vi "thcd_400_control_1.vi"() -> ()   [LabVIEW 2019]
uses:
  thcd_controls/ctrl_chn_thcd.ctl
  thcd_controls/ctrl_sms_thcd.ctl
  <vilib>/Utility/file.llb/Write Delimited Spreadsheet (DBL).vi
  thcd_commands/thcd_set_samp.vi
panel:
  out "Sensor data":cluster{cluster{"X":dbl, "Y":dbl}[]}[](graph)
  out "thcd_st":bool
  out "thcd_res_msg":string
  in  "thcd_val":dbl min=0.0 max=100.0 step=1.0 format="%#.6g"
  in  "milliseconds to wait":u32
  out "thcd_res_4":T2
  out "thcd_res_3":T2
  out "thcd_res_2":T2
  out "thcd_res_1":T2
  in  "getstat":bool
  in  "set":bool
  in  "read":bool
  out "res_val 3":dbl
  out "res_val 2":dbl
  out "res_val":dbl
  in  "Baud_rate":u32(ring)=19200 items=["9.6KHz"=9600, "19.2KHz"=19200]
  in  "thcd_visa":refnum<visa-resource-name>
  in  "Init Devices":bool
  in  "Exit":bool
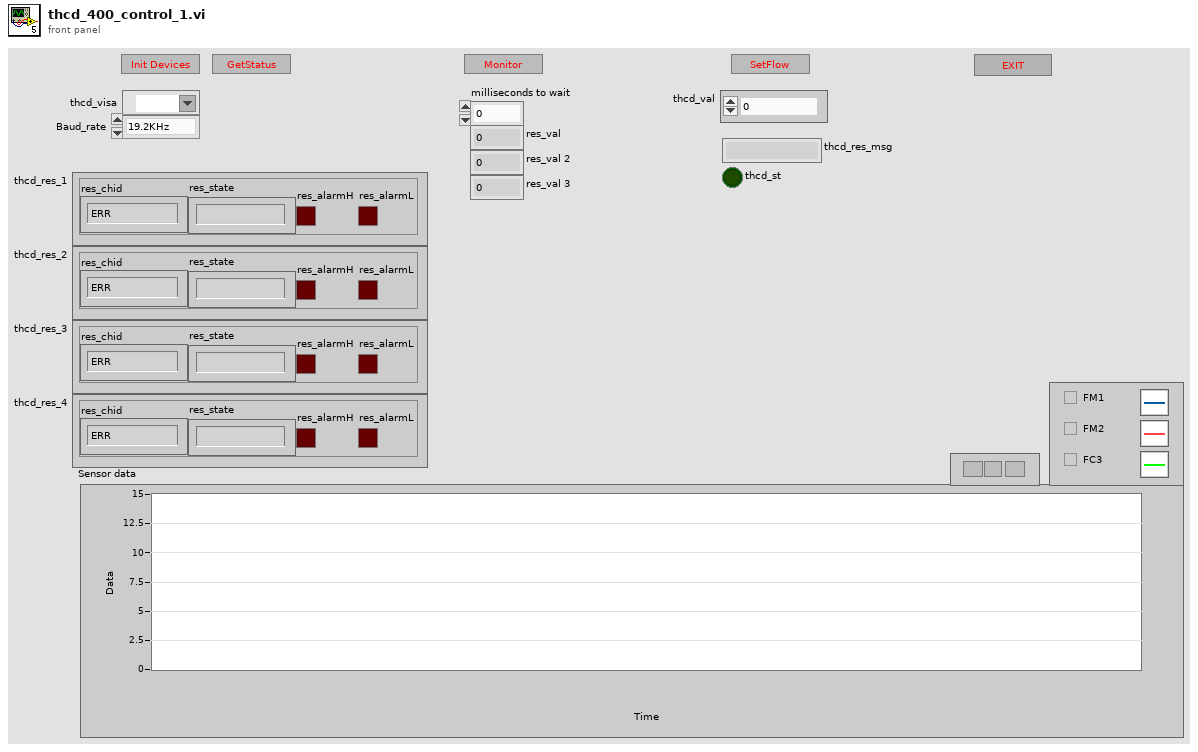
[diagram p1: front panel]
types:
  T1 = typedef "ctrl_chn_thcd.ctl" = enum8{"ERR", "1", "2", "3", "4"}
  T2 = cluster{"res_chid":T1, "res_state":string, "res_alarmH":bool, "res_alarmL":bool}
  T3 = typedef "ctrl_sms_thcd.ctl" = enum16{"idle", "init", "exit", "read", "set", "getstat"}
  T4 = enum16{"SetPoint", "AlarmH", "AlarmL", "Multiplier", "CalibValue"}
  T5 = cluster{"res_chid":T1, "res_val":dbl, "res_uom":string, "res_gid":string}[]
  T6 = cluster{"res_chid":T1, "res_val":dbl, "res_uom":string, "res_gid":string}
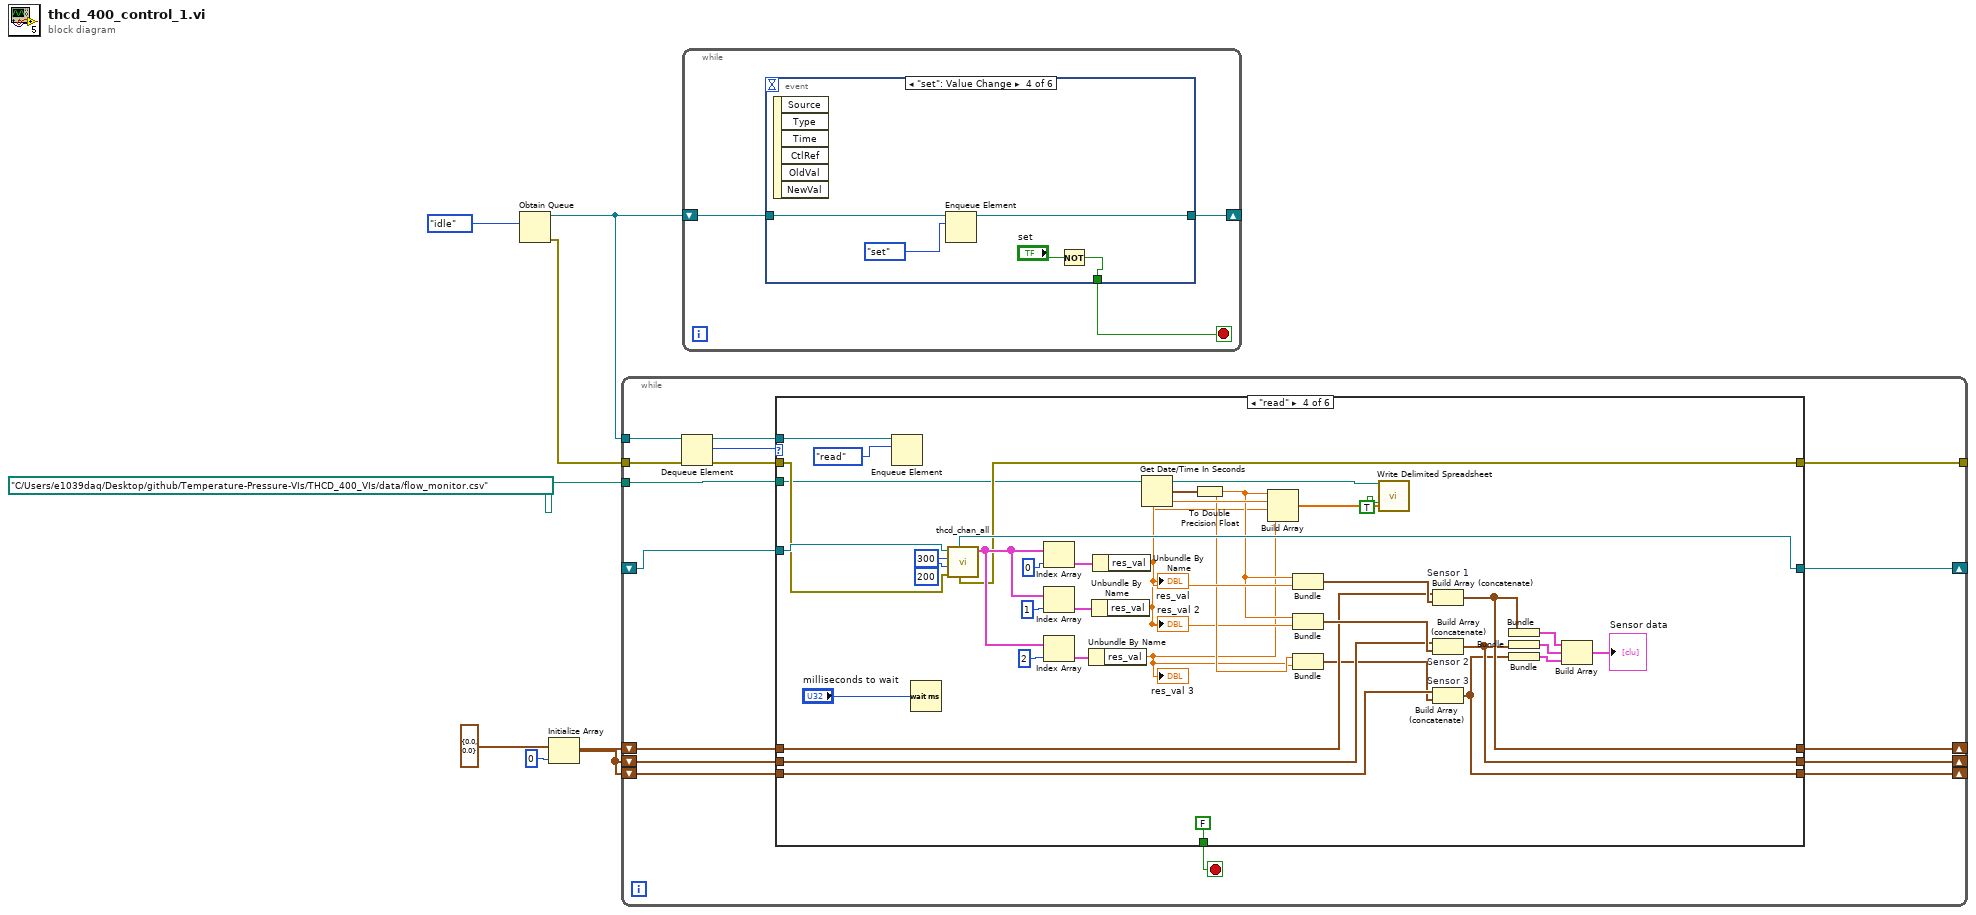
[diagram p0: block diagram]
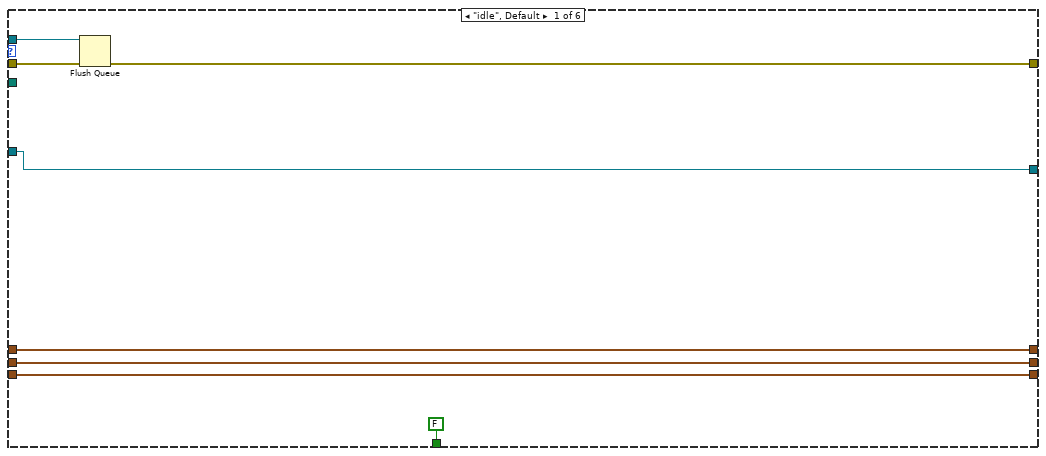
[diagram p2: hidden frame]
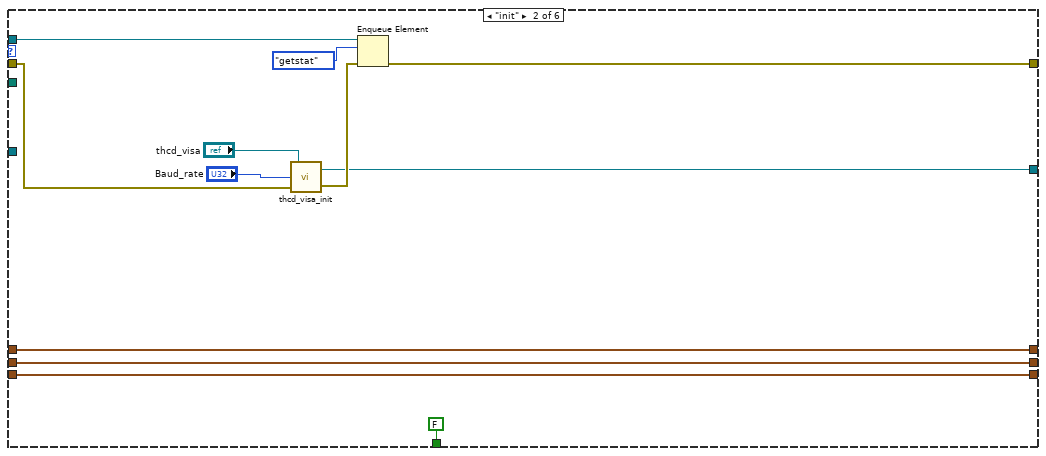
[diagram p3: hidden frame]
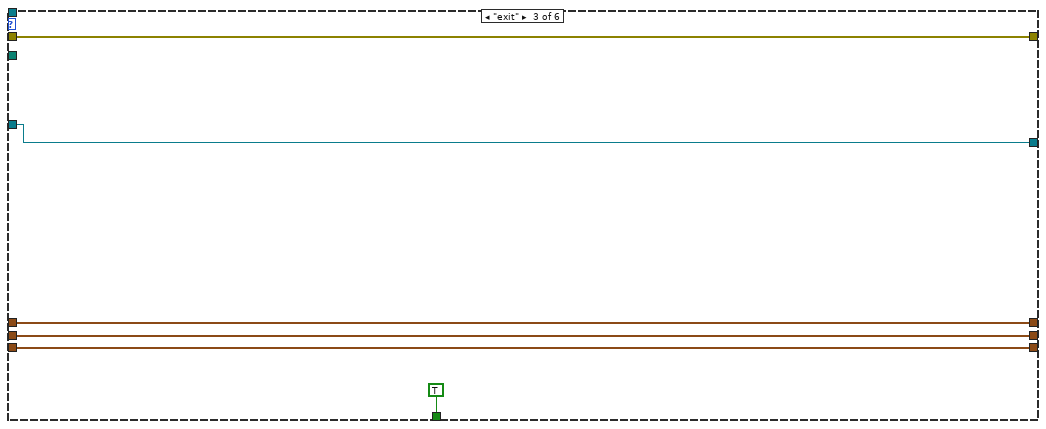
[diagram p4: hidden frame]
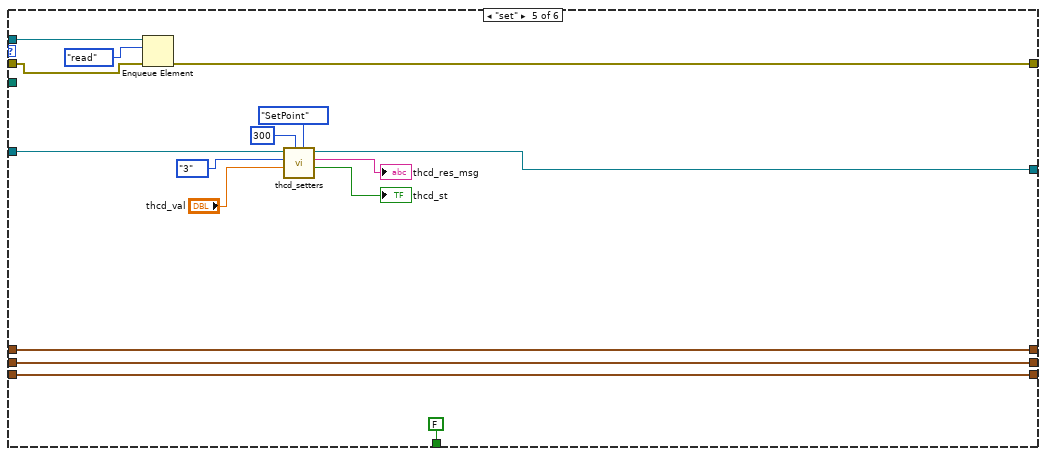
[diagram p5: hidden frame]
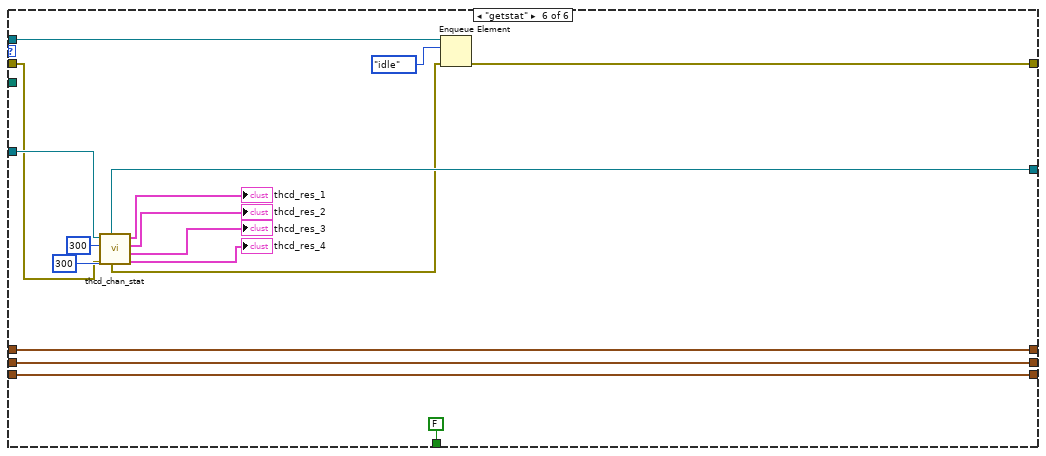
[diagram p6: hidden frame]
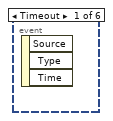
[diagram p7: hidden frame]
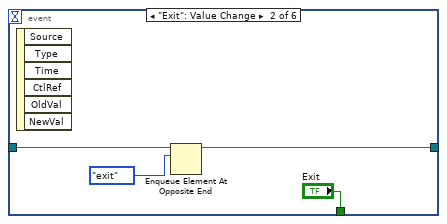
[diagram p8: hidden frame]
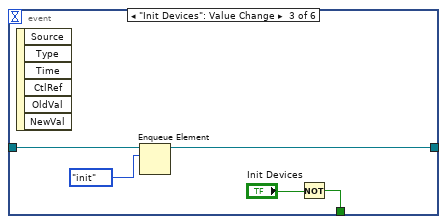
[diagram p9: hidden frame]
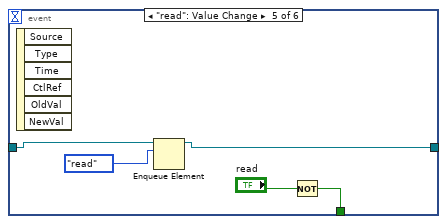
[diagram p10: hidden frame]
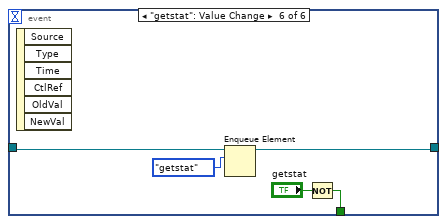
[diagram p11: hidden frame]
diagram:
  n1 = Obtain Queue(element data type=ctrl_sms_thcd."idle" ("Enum")) -> (queue out=w6:refnum<queue>, error out=w5:errorcluster)  [unwired: 4 in, 1 out]
  n2 = Initialize Array(cluster{"X":dbl, "Y":dbl} {"X"=0.0, "Y"=0.0}, 0 ("dimension size")) -> (w1:cluster{"X":dbl, "Y":dbl}[])
  n3 = while {
    tunnel: w5 -> [w21]
    tunnel: [w18] -> _
    tunnel: w6 -> [w22]
    shift-right: [w16] -> _
    shift-left: _ -> [w15]
    tunnel: path "C:/Users/e1039daq/Desktop/github/Temperature-Pressure-VIs/THCD_400_VIs/data/flow_monitor.csv" ("file path (dialog if empty)") -> [w14]
    shift-right: [w10] -> _
    shift-left: w1 -> [w13]
    shift-right: [w9] -> _
    shift-left: w1 -> [w12]
    shift-right: [w8] -> _
    shift-left: w1 -> [w11]
    stop <- w23 stop-if-true
    n4 = Dequeue Element(queue=w22, error in (no error)=w21) -> (queue out=w17:refnum<queue>, element=w20:T3, error out=w19:errorcluster)  [unwired: 1 in, 1 out]
    n5 = case shown="\"read\"" w20 {
      tunnel: w17 -> [w30 w39 _ w71 w101 w110]
      tunnel: [FALSE FALSE TRUE FALSE FALSE FALSE] -> w23
      tunnel: w19 -> [w29 w40 w48 w86 w100 w116]
      tunnel: [w28 w36 w48 w75 w99 w108] -> w18
      tunnel: [w27 w35 w47 w83 w97 w119] -> w16
      tunnel: w15 -> [w27 _ w47 w87 w98 w120]
      tunnel: w14 -> [_ _ _ w67 _ _]
      tunnel: w13 -> [w26 w34 w46 w57 w90 w106]
      tunnel: w12 -> [w25 w33 w45 w56 w89 w105]
      tunnel: w11 -> [w24 w32 w44 w55 w88 w104]
      tunnel: [w26 w34 w46 w52 w90 w106] -> w10
      tunnel: [w25 w33 w45 w51 w89 w105] -> w9
      tunnel: [w24 w32 w44 w50 w88 w104] -> w8
      frame "idle", Default {
        n6 = Flush Queue(queue=w30, error in (no error)=w29) -> (error out=w28:errorcluster)  [unwired: 2 out]
      }
      frame "init" {
        n7 = call "thcd_visa_init.vi"("err_in"=w40, "Serial Settings:Baud Rate"="Baud_rate", "thcd_visa"="thcd_visa") -> ("err_out"=w37:errorcluster, "thcd_visa"=w35:refnum<visa-resource-name>)
        n8 = Enqueue Element(queue=w39, element=ctrl_sms_thcd."getstat", error in (no error)=w37) -> (error out=w36:errorcluster)  [unwired: 1 in, 2 out]
      }
      frame "exit" {
      }
      frame "read" {
        n9 = Enqueue Element(queue=w71, element=ctrl_sms_thcd."read") -> ()  [unwired: 2 in, 3 out]
        n10 = Wait (ms)(milliseconds to wait="milliseconds to wait") -> ()  [unwired: 1 out]
        n11 = call "thcd_chan_all.vi"("err_in"=w86, "thcd_b2r"=u32 200, "thcd_delay"=u32 300, "thcd_visa"=w87) -> ("thcd_res"=w76:T5, "err_out"=w75:errorcluster, "thcd_visa"=w83:refnum<visa-resource-name>)  [unwired: 3 in, 2 out]
        n12 = Index Array(array=w76, index=0) -> (element=w81:T6)
        n13 = Index Array(array=w76, index=1) -> (element=w80:T6)
        n14 = Index Array(array=w76, index=2) -> (element=w79:T6)
        n15 = Unbundle By Name(w79) -> ("res_val"=w58:dbl)
        "res_val 3" <- w58
        n16 = Unbundle By Name(w80) -> ("res_val"=w59:dbl)
        "res_val 2" <- w59
        n17 = Unbundle By Name(w81) -> ("res_val"=w61:dbl)
        "res_val" <- w61
        n18 = Get Date/Time In Seconds() -> (seconds since 1Jan1904=w70:timestamp)
        n19 = To Double Precision Float(number=w70) -> (double precision float=w60:dbl)
        n20 = Build Array(w60, w61, w59, w58) -> (w69:dbl[])
        n21 = Bundle(w60, "res_val"=w61) -> (w66:cluster{dbl, "res_val":dbl})  [unwired: 1 in]
        n22 = Bundle(w60, "res_val"=w59) -> (w62:cluster{dbl, "res_val":dbl})  [unwired: 1 in]
        n23 = Bundle(w60, "res_val"=w58) -> (w54:cluster{dbl, "res_val":dbl})  [unwired: 1 in]
        n24 = call-poly <vilib>:"Write Delimited Spreadsheet.vi"("file path (dialog if empty)"=w67, "1D data"=w69, "append to file? (new file:F)"=TRUE ("append to file? (F)")) -> ()  [unwired: 11 in, 2 out]
        n25 = Build Array (concatenate) "Sensor 1"(w57, w66) -> (w52:cluster{"X":dbl, "res_val":dbl}[])
        n26 = Build Array (concatenate) "Sensor 2"(w56, w62) -> (w51:cluster{"X":dbl, "res_val":dbl}[])
        n27 = Build Array (concatenate) "Sensor 3"(w55, w54) -> (w50:cluster{"X":dbl, "res_val":dbl}[])
        n28 = Bundle(w52) -> (w65:cluster{cluster{"X":dbl, "res_val":dbl}[]})  [unwired: 1 in]
        n29 = Bundle(w51) -> (w63:cluster{cluster{"X":dbl, "res_val":dbl}[]})  [unwired: 1 in]
        n30 = Bundle(w50) -> (w53:cluster{cluster{"X":dbl, "res_val":dbl}[]})  [unwired: 1 in]
        n31 = Build Array(w65, w63, w53) -> (→"Sensor data":cluster{cluster{"X":dbl, "res_val":dbl}[]}[])
      }
      frame "set" {
        n32 = Enqueue Element(queue=w101, element=ctrl_sms_thcd."read", error in (no error)=w100) -> (error out=w99:errorcluster)  [unwired: 1 in, 2 out]
        n33 = call-poly "thcd_setters.vi"("thcd_com"=T4."SetPoint", "thcd_delay"=u32 300, "thcd_val"="thcd_val", "thcd_ch"=ctrl_chn_thcd."3", "thcd_visa"=w98) -> ("thcd_st"=→"thcd_st":bool, "thcd_res_msg"=→"thcd_res_msg":string, "thcd_visa"=w97:refnum<visa-resource-name>)  [unwired: 1 in, 1 out]
      }
      frame "getstat" {
        n34 = call "thcd_chan_stat.vi"("err_in"=w116, "thcd_b2r"=u32 300, "thcd_delay"=u32 300, "thcd_visa"=w120) -> ("thcd_res_4"=→"thcd_res_4":T2, "thcd_res_3"=→"thcd_res_3":T2, "thcd_res_2"=→"thcd_res_2":T2, "thcd_res_1"=→"thcd_res_1":T2, "err_out"=w109:errorcluster, "thcd_visa"=w119:refnum<visa-resource-name>)  [unwired: 2 out]
        n35 = Enqueue Element(queue=w110, element=ctrl_sms_thcd."idle", error in (no error)=w109) -> (error out=w108:errorcluster)  [unwired: 1 in, 2 out]
      }
    }
  }
  n36 = while {
    shift-right: [w122] -> _
    shift-left: w6 -> [w123]
    stop <- w121 stop-if-true
    n37 = event shown="[3] \"set\": Value Change" {
      selector: _ -> [_ _ _ _ _ _]
      dyn-events: _ -> [_ _ _ _ _ _]
      timeout: _ -> [_ _ _ _ _ _]
      tunnel: w123 -> [_ w127 w132 w134 w140 w145]
      tunnel: [_ w126 w131 w133 w139 w144] -> w122
      tunnel: [_ "Exit" w128 w136 w141 w146] -> w121
      event Timeout {
        n38 = event-data() -> ()  [unwired: 1 in, 3 out]
      }
      event "Exit": Value Change {
        n39 = event-data() -> ()  [unwired: 1 in, 6 out]
        n40 = Enqueue Element At Opposite End(queue=w127, element=ctrl_sms_thcd."exit" ("Enum")) -> (queue out=w126:refnum<queue>)  [unwired: 2 in, 2 out]
      }
      event "Init Devices": Value Change {
        n41 = event-data() -> ()  [unwired: 1 in, 6 out]
        n42 = Enqueue Element(queue=w132, element=ctrl_sms_thcd."init") -> (queue out=w131:refnum<queue>)  [unwired: 2 in, 2 out]
        n43 = Not(x="Init Devices") -> (.not. x?=w128:bool)
      }
      event "set": Value Change {
        n44 = event-data() -> ()  [unwired: 1 in, 6 out]
        n45 = Enqueue Element(queue=w134, element=ctrl_sms_thcd."set" ("Enum")) -> (queue out=w133:refnum<queue>)  [unwired: 2 in, 2 out]
        n46 = Not(x="set") -> (.not. x?=w136:bool)
      }
      event "read": Value Change {
        n47 = event-data() -> ()  [unwired: 1 in, 6 out]
        n48 = Enqueue Element(queue=w140, element=ctrl_sms_thcd."read" ("Enum")) -> (queue out=w139:refnum<queue>)  [unwired: 2 in, 2 out]
        n49 = Not(x="read") -> (.not. x?=w141:bool)
      }
      event "getstat": Value Change {
        n50 = event-data() -> ()  [unwired: 1 in, 6 out]
        n51 = Enqueue Element(queue=w145, element=ctrl_sms_thcd."getstat") -> (queue out=w144:refnum<queue>)  [unwired: 2 in, 2 out]
        n52 = Not(x="getstat") -> (.not. x?=w146:bool)
      }
    }
  }
